vi "CRC16校验IsRight.vi"(2 "含检验码数据长度":u16, 3 "输入数据":u8[](array[numeric])) -> (0 "原始数据":string, 1 "布尔":bool)   [LabVIEW 2015]
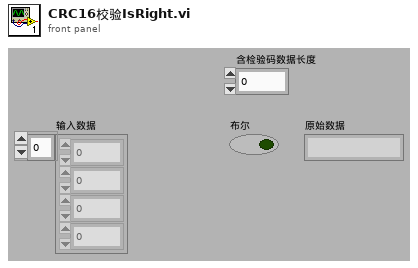
[diagram p1: front panel]
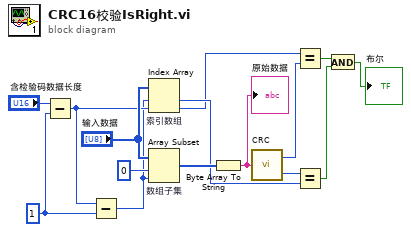
[diagram p0: block diagram]
diagram:
  w2 = 1 ("y")
  n1 = Subtract(x="含检验码数据长度", y=w2) -> (x-y=w3:i32)
  n2 = Subtract(x=w3, y=w2) -> (x-y=w1:i32)
  n3 = Index Array "索引数组"(array="输入数据", index #1=w1, index #2=w3) -> (element #1=w12:u8, element #2=w9:u8)
  n4 = Array Subset "数组子集"(array="输入数据", index=0 ("索引"), length=w1) -> (w13:u8[])
  n5 = Byte Array To String(unsigned byte array=w13) -> (string=w15:string)
  "原始数据" <- w15
  n6 = call "CRC.vi"("输入字符串"=w15) -> ("CRC高8位"=w10:u8, "CRC低8位"=w11:u8)
  n7 = Equal?(x=w9, y=w10) -> (x = y?=w7:bool)
  n8 = Equal?(x=w11, y=w12) -> (x = y?=w8:bool)
  n9 = And(x=w7, y=w8) -> (x .and. y?=→"布尔":bool)
